vi "Done.vi"(8 "error in (no error)":errorcluster, 11 "Network Sink in":refnum<class "Network Sink.lvclass">) -> (0 "error out":errorcluster)   [LabVIEW 2019, in "Network Sink.lvlib" / "Network Sink.lvclass"]
doc: "--\nCopyright © 2017 Composed SystemsI All rights reserved.\n\nAuthor: Jon McBee <jon.mcbee@composed.io>\n\nThis library is provided \"AS IS\" ,WITHOUT WARRANTIES OR\nCONDITIONS OF ANY KIND, either express or implied.\n\nComposed Systems -- composed.io\n\nStream 0.0.1.1\nJon McBee - Composed Systems\nCopyright (c) 2017, Composed Systems"
uses:
  <vilib>/gpm_packages/@cs/event-logger/Source/Network Sink/Network Sink/Network Sink.lvclass
  <vilib>/gpm_packages/@cs/event-logger/Source/Network Sink/Network Sink/Network Sink.lvclass/Network Sink.ctl
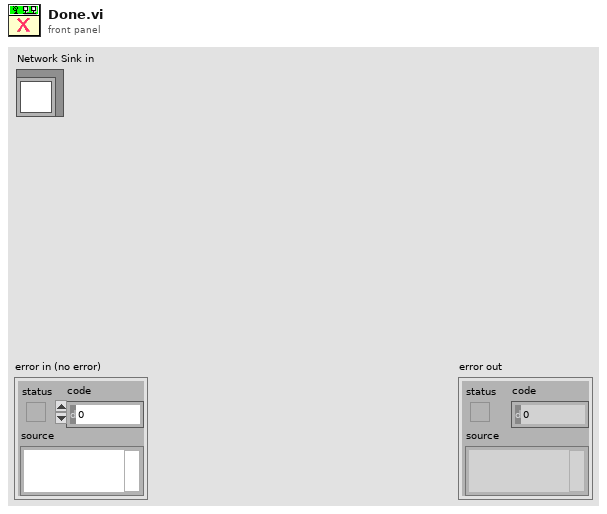
[diagram p1: front panel]
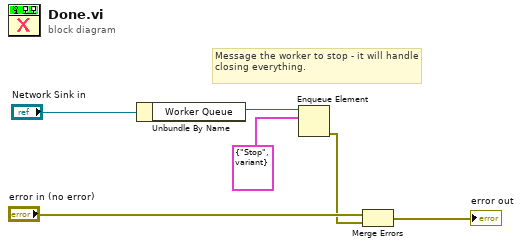
[diagram p0: block diagram]
diagram:
  # "Message the worker to stop - it will handle closing everything."
  n1 = Unbundle By Name("Network Sink in") -> ("Worker Queue"=w4:refnum<queue>)
  n2 = Enqueue Element(queue=w4, element=cluster{"Message":string, "Data":variant} {"Message"="Stop", "Data"=variant}) -> (error out=w1:errorcluster)  [unwired: 2 in, 2 out]
  n3 = Merge Errors("error in (no error)", w1) -> (→"error out":errorcluster)
